vi "Create Pattern BIN.vi"(8 "error in (no error)":errorcluster, 11 "BML_Root in":refnum<class "BML_Root.lvclass">) -> (0 "error out":errorcluster, 3 "BML_Root out":refnum<class "BML_Root.lvclass">)   [LabVIEW 2016, in "BML_Root.lvclass"]
uses:
  BML_Root.lvclass
  BML_Root.lvclass/BML_Root.ctl
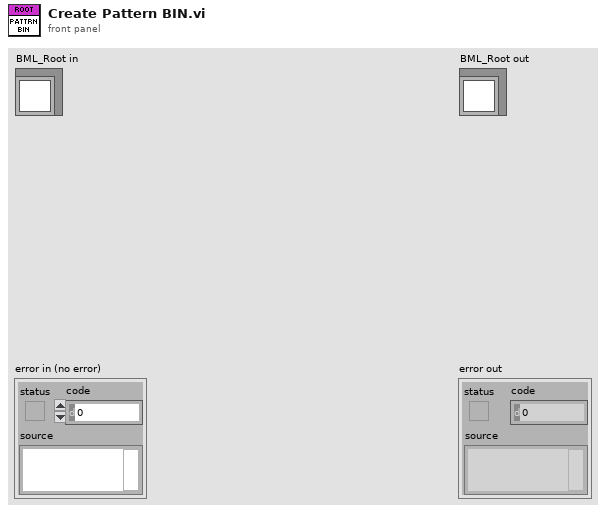
[diagram p1: front panel]
types:
  T1 = enum16{"open", "replace", "create", "open or create", "replace or create", "replace or create with confirmation"}
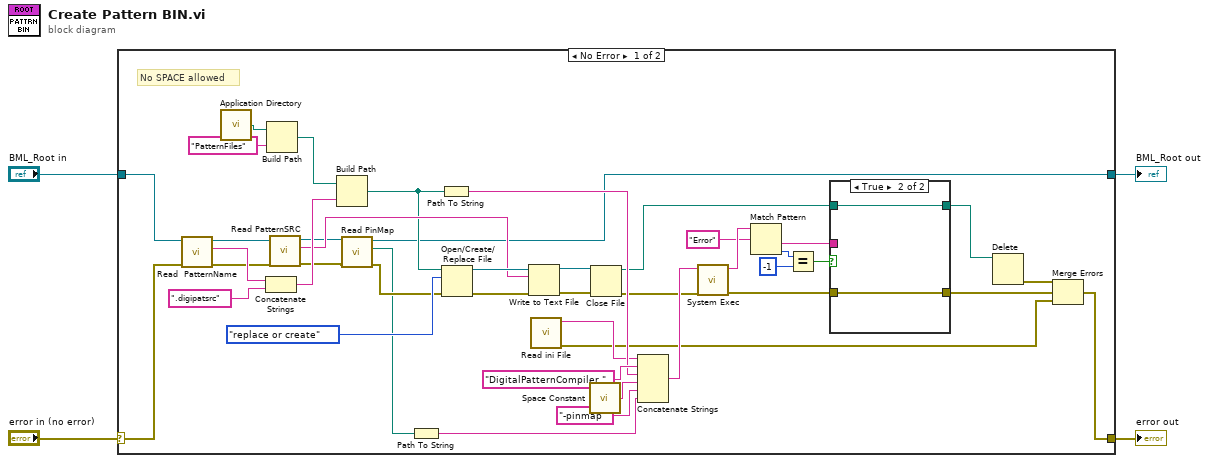
[diagram p0: block diagram]
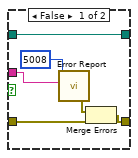
[diagram p2: hidden frame]
diagram:
  n1 = case shown="No Error" "error in (no error)" {
    selector: "error in (no error)" -> [w46 w57]
    tunnel: [w16 w57] -> w3
    tunnel: [w15 w56] -> w1
    tunnel: "BML_Root in" -> [w47 w56]
    frame No Error {
      # "No SPACE allowed"
      n2 = call "Read  PatternName.vi"("error in (no error)"=w46, "BML_Root in"=w47) -> ("error out"=w40:errorcluster, "PatternName"=w45:string, "BML_Root out"=w39:refnum<class "BML_Root.lvclass">)  [unwired: 7 in]
      n3 = call <vilib>:"Application Directory.vi"() -> ("Application Directory"=w11:path)
      n4 = Concatenate Strings(w45, ".digipatsrc" ("string")) -> (w43:string)
      n5 = Build Path(base path=w11, name or relative path="PatternFiles") -> (appended path=w9:path)
      n6 = call "Read PatternSRC.vi"("error in (no error)"=w40, "BML_Root in"=w39) -> ("error out"=w29:errorcluster, "PatternSRC"=w38:string, "BML_Root out"=w30:refnum<class "BML_Root.lvclass">)  [unwired: 7 in]
      n7 = Build Path(base path=w9, name or relative path=w43) -> (appended path=w35:path)
      n8 = call "Read PinMap.vi"("error in (no error)"=w29, "BML_Root in"=w30) -> ("error out"=w28:errorcluster, "PinMap"=w27:path, "BML_Root out"=w15:refnum<class "BML_Root.lvclass">)  [unwired: 7 in]
      n9 = Path To String(path=w27) -> (string=w26:string)
      n10 = Path To String(path=w35) -> (string=w34:string)
      n11 = Open/Create/Replace File(file path (use dialog)=w35, error in=w28, operation (0:open)=T1."replace or create") -> (refnum out=w41:refnum<file>, error out=w37:errorcluster)  [unwired: 3 in, 1 out]
      n12 = Write to Text File(file (use dialog)=w41, text=w38, error in=w37) -> (refnum out=w14:refnum<file>, error out=w13:errorcluster)  [unwired: 1 in, 1 out]
      n13 = call "Read ini File.vi"() -> ("error out"=w7:errorcluster, "value"=w31:string)  [unwired: 10 in]
      n14 = call <vilib>:"Space Constant.vi"() -> ("String"=w33:string)
      n15 = Close File(refnum=w14, error in=w13) -> (path=w6:path, error out=w12:errorcluster)
      n16 = Concatenate Strings(w31, "DigitalPatternCompiler " ("string"), w34, w33, "-pinmap " ("string"), w26) -> (w25:string)
      n17 = call <vilib>:"System Exec.vi"("error in (no error)"=w12, "command line"=w25) -> ("error out"=w18:errorcluster, "standard output"=w24:string)  [unwired: 6 in, 2 out]
      n18 = Match Pattern(string=w24, regular expression="Error") -> (after substring=w19:string, offset past match=w22:i32)  [unwired: 1 in, 2 out]
      n19 = Equal?(x=w22, y=-1) -> (x = y?=w20:bool)
      n20 = case shown="True" w20 {
        tunnel: w19 -> [w53 _]
        tunnel: w18 -> [w51 w55]
        tunnel: [w49 w55] -> w17
        tunnel: w6 -> [w48 w54]
        tunnel: [w48 w54] -> w5
        frame False {
          n21 = call "Error Report.vi"("Additional info"=w53, "Error Code"=i16 5008) -> ("error out"=w52:errorcluster)  [unwired: 9 in]
          n22 = Merge Errors(w52, w51) -> (w49:errorcluster)
        }
        frame True {
        }
      }
      n23 = Delete(path (use dialog)=w5) -> (error out=w8:errorcluster)  [unwired: 4 in, 2 out]
      n24 = Merge Errors(w8, w17, w7) -> (w16:errorcluster)
    }
    frame Error {
    }
  }
  "error out" <- w3
  "BML_Root out" <- w1
